vi "Read QR Code.vi"() -> ()   [LabVIEW 2014]
doc: "This example illustrates how to use the Read QR Code VI. There are several types of QR codes that are supported including Micro, Model 1 and Model 2, as well as various cell shapes and barcode shapes."
uses:
  <vilib>/vision/Instrument.llb/QR Code Description Options.ctl
  <vilib>/vision/Instrument.llb/Data Matrix Polarity.ctl
  <vilib>/vision/Instrument.llb/QR Code Model Type.ctl
  <vilib>/vision/Instrument.llb/QR Code Search Options.ctl
  <vilib>/vision/Instrument.llb/Demodulation Mode.ctl
  <vilib>/vision/Instrument.llb/Cell Sample Size.ctl
  <vilib>/vision/Instrument.llb/Cell Filter Mode.ctl
  <vilib>/vision/NI_Vision_Development_Module.lvlib
panel:
  out "Read Time (ms)":dbl format="%.2f"
  out "Data":string
  out "Image":T1(plugin-control)
  # "Overview: Demonstrate the reading of QR Codes.\nRequirements: Vision Development Module.\nInstructions: Run the VI."
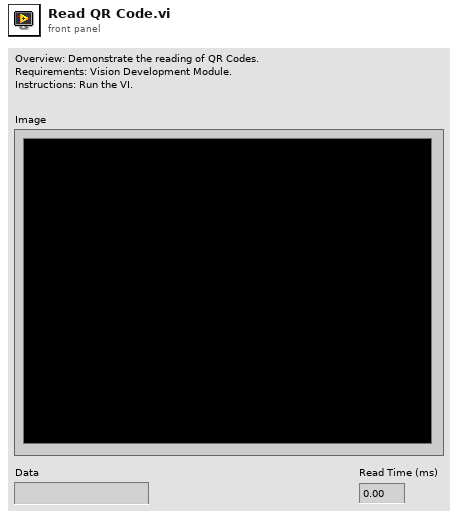
[diagram p1: front panel]
types:
  T1 = typedef "IMAQ Image.ctl" = refnum<image>
  T2 = typedef "QR Code Search Options.ctl" = cluster{"Rotation Mode":enum32{"Unlimited", "0 Degrees", "90 Degrees", "180 Degrees", "270 Degrees"}, "Skip Location?":bool, "Edge Threshold":u32, "Demodulation Mode":T3, "Cell Sample Size":T4, "Cell Filter Mode":T5, "Skew Degrees Allowed":u32}
  T3 = typedef "Demodulation Mode.ctl" = i32
  T4 = typedef "Cell Sample Size.ctl" = i32
  T5 = typedef "Cell Filter Mode.ctl" = i32
  T6 = typedef "QR Code Description Options.ctl" = cluster{"Matrix Size (cells)":i32, "Barcode Polarity":T7, "Mirror Mode":i32, "QR Model":T8}
  T7 = typedef "Data Matrix Polarity.ctl" = i32
  T8 = typedef "QR Code Model Type.ctl" = i32
  T9 = typedef "QR Code Report.ctl" = cluster{"Found?":bool, "Data":string, "Bounding Box":cluster{"x":sgl, "y":sgl}[], "Errors Corrected":u32, "Dimensions (Rows/Cols)":u32, "Version":u32, "QR Model":T8, "Stream Mode":T10, "Barcode Polarity":T7, "Mirrored?":bool, "Append Stream Position":u32, "Size of Append Stream":u32, "First EAN-128 ID":i32, "First Alternate Language ID":i32, "Append Stream ID":u32, "Minimum Edge Strength":u32, "Demodulation Mode":T3, "Cell Sample Size":T4, "Cell Filter Mode":T5}
  T10 = typedef "QR Code Stream Mode Type.ctl" = i32
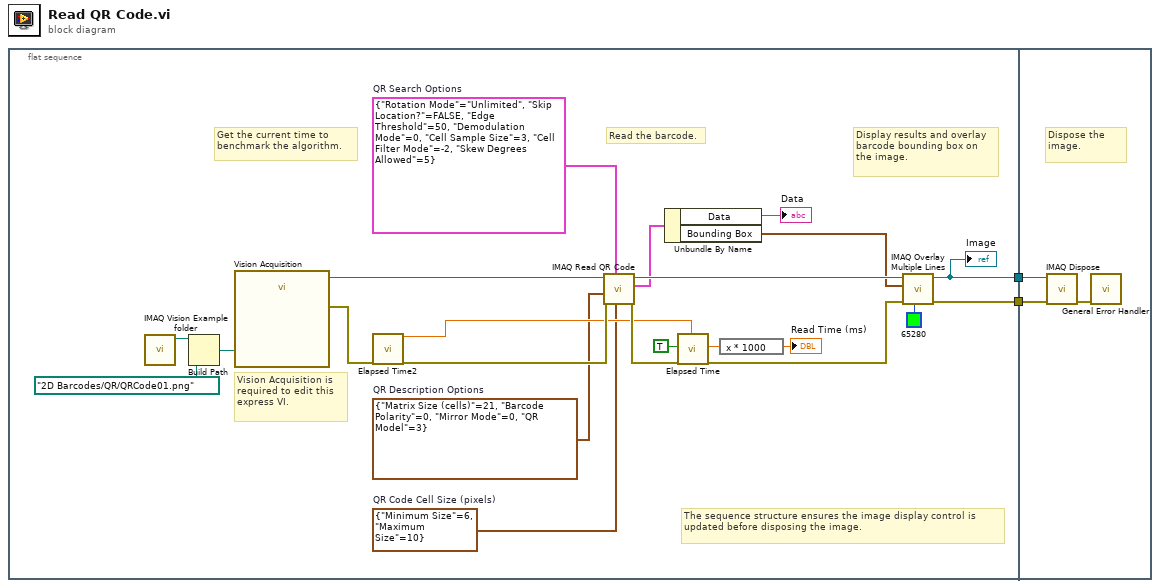
[diagram p0: block diagram]
diagram:
  n1 = flat-sequence {
    tunnel: [w9] -> w2
    tunnel: [w24] -> w1
    tunnel: w2 -> [w26]
    tunnel: w1 -> [w25]
    frame #0 {
      w7 = T2 {"Rotation Mode"=enum."Unlimited", "Skip Location?"=FALSE, "Edge Threshold"=50, "Demodulation Mode"=0, "Cell Sample Size"=3, "Cell Filter Mode"=-2, "Skew Degrees Allowed"=5}  # QR Search Options
      w6 = T6 {"Matrix Size (cells)"=21, "Barcode Polarity"=0, "Mirror Mode"=0, "QR Model"=3}  # QR Description Options
      w5 = cluster{"Minimum Size":u32, "Maximum Size":u32} {"Minimum Size"=6, "Maximum Size"=10}  # QR Code Cell Size (pixels)
      # "The sequence structure ensures the image display control is updated before disposing the image."
      # "Vision Acquisition is required to edit this express VI."
      # "Read the barcode."
      # "Get the current time to benchmark the algorithm."
      # "Display results and overlay barcode bounding box on the image."
      n2 = call "IMAQ Vision Example folder.vi"() -> ("Example Image Path"=w23:path)  [unwired: 11 in]
      n3 = Build Path(base path=w23, name or relative path=path "2D Barcodes/QR/QRCode01.png" ("path out")) -> (appended path=w13:path)
      n4 = call "Vision Acquisition"("Image Path"=w13) -> ("Image Out"=w20:T1, "error out"=w16:errorcluster)  [unwired: 25 in]
      n5 = call "Elapsed Time2"("error in (no error)"=w16) -> ("Present (s)"=w10:dbl, "error out"=w15:errorcluster)  [unwired: 11 in, 6 out]
      n6 = call "IMAQ Read QR Code"("QR Code Cell Size (pixels)"=w5, "QR Search Options"=w7, "error in (no error)"=w15, "QR Description Options"=w6, "Image"=w20) -> ("error out"=w12:errorcluster, "QR Code Report"=w17:T9, "Image (duplicate)"=w18:T1)  [unwired: 3 in, 1 out]
      n7 = Unbundle By Name(w17) -> ("Data"=→"Data":string, "Bounding Box"=w4:cluster{"x":sgl, "y":sgl}[])
      n8 = call "Elapsed Time"("Reset"=TRUE, "error in (no error)"=w12, "Set Start Time (s)"=w10) -> ("Elapsed Time (s)"=w21:dbl, "error out"=w11:errorcluster)  [unwired: 9 in, 6 out]
      n9 = expression code="x * 1000"(w21) -> (→"Read Time (ms)":dbl)
      n10 = call "IMAQ Overlay Multiple Lines"("Color"=u32 65280, "error in (no error)"=w11, "Line End Points"=w4, "Image"=w18) -> ("error out"=w24:errorcluster, "Image Out"=w9:T1)  [unwired: 6 in]
      "Image" <- w9
    }
    frame #1 {
      # "Dispose the image."
      n11 = call "IMAQ Dispose"("Image"=w26, "error in (no error)"=w25) -> ("error out"=w27:errorcluster)  [unwired: 4 in]
      n12 = call <vilib>:"General Error Handler.vi"("error in (no error)"=w27) -> ()  [unwired: 10 in, 5 out]
    }
  }
